vi "InTurtleMode.vi"(9 "MaxStayForce":dbl, 10 "WindSpeed (m/s)":dbl, 11 "HindbrainEmergencySailOverrideOn":bool) -> (3 "InTurtleMode?":bool)   [LabVIEW 2012]
doc: "This VI is intended to sense the Hindbrain emergency mode and call a Midbrain emergency if the Hindbrain calls a number of emergencies in a short period of time. If the Hindbrain is frequently letting out the sails due to excessive stress, the Midbrain should put the boat in turtle mode for some medium length of time, maybe a minute or two, and determine whether to come out of turtle mode based on whether both the wind speed and stay forces are in safe bounds.\n\nThis will need some sort of relative time reference, for two reasons. First, it will be needed in order to say \"how many HB emergencies have happened in the last 5 minutes?\". Second, it will be needed in order to say \"I've called a MB emergency for 45 seconds, I'll return TRUE every time I am queried in the next 15 seconds\".\n\nEric Schneider, Jan. 2014"
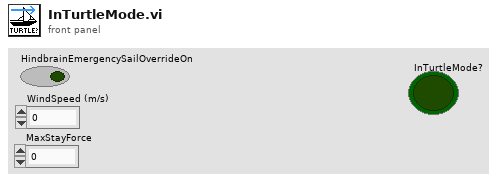
[diagram p1: front panel]
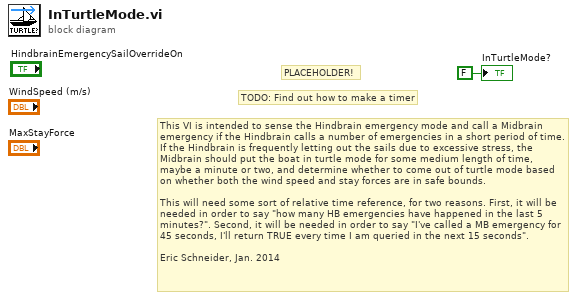
[diagram p0: block diagram]
diagram:
  # "TODO: Find out how to make a timer"
  # "PLACEHOLDER!"
  # "This VI is intended to sense the Hindbrain emergency mode and call a Midbrain emergency if the Hindbrain calls a number of emergencies in a short period of time. If the Hindbrain is frequently letting out the sails due to excessive stress, the Midbrain should put the boat in turtle mode for some medium length of time, maybe a minute or two, and determine whether to come out of turtle mode based on whether both the wind speed and stay forces are in safe bounds.\n\nThis will need some sort of relative time reference, for two reasons. First, it will be needed in order to say \"how many HB emergencies have happened in the last 5 minutes?\". Second, it will be needed in order to say \"I've called a MB emergency for 45 seconds, I'll return TRUE every time I am queried in the next 15 seconds\".\n\nEric Schneider, Jan. 2014"
  "InTurtleMode?" <- FALSE ("InTurtleMode?")
